vi "Remove Minor Frames.vi"(8 "error in (no error)":errorcluster, 10 "Minor Frame IDs":string[](array[string]), 11 "Major Frame in":refnum<class "Major Frame.lvclass">) -> (0 "error out":errorcluster, 3 "Major Frame out":refnum<class "Major Frame.lvclass">)   [LabVIEW 2020, in "BCI-1553 API.lvlib" / "Major Frame.lvclass"]
doc: "Removes a collection of Minor Frames from this Major Frame. These removed Minor Frames are no longer available to the Major Frame Schedule. The calling code must supply a new Schedule if the existing Schedule depends on a removed Minor Frame."
uses:
  Major Frame.lvclass
  Major Frame.lvclass/Major Frame.ctl
  Dependencies/Registry/Registry.lvclass/Registry.ctl
  Dependencies/Registry/Registry.lvclass
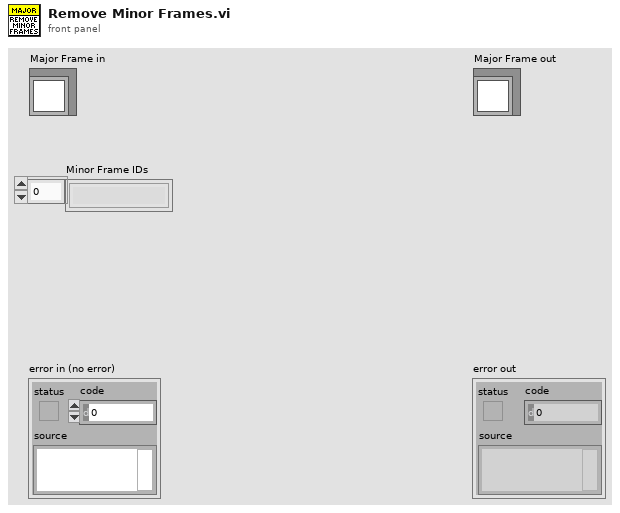
[diagram p1: front panel]
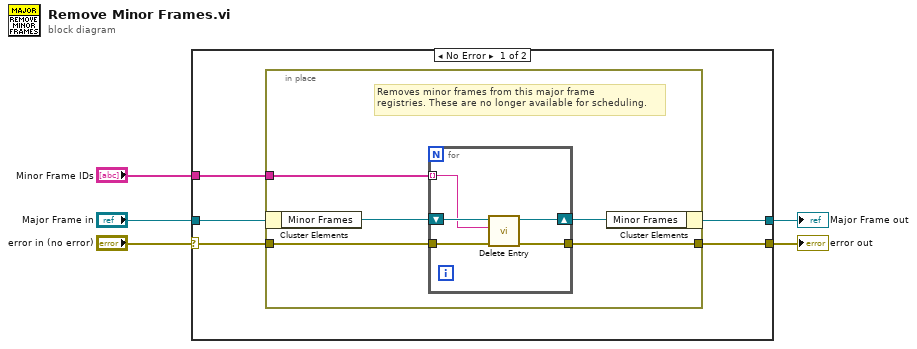
[diagram p0: block diagram]
diagram:
  n1 = case shown="No Error" "error in (no error)" {
    selector: "error in (no error)" -> [w7 w22]
    tunnel: [w8 w22] -> w3
    tunnel: [w9 w21] -> w2
    tunnel: "Major Frame in" -> [w10 w21]
    tunnel: "Minor Frame IDs" -> [w6 _]
    frame No Error {
      n2 = in-place {
        in-place-border: [w12] -> w8
        in-place-border: w7 -> [w14]
        in-place-border: w6 -> [w13]
        # "Removes minor frames from this major frame\nregistries. These are no longer available for scheduling."
        n3 = in-place-cluster #1(w10) -> ("Minor Frames"=w15:refnum<class "Registry.lvclass">)
        n4 = for {
          shift-right: [w17] -> w11
          shift-left: w15 -> [w20]
          tunnel: w14 -> [w19]
          tunnel: w13 -> [w18] mode=indexing
          tunnel: [w16] -> w12
          n5 = call "Delete Entry.vi"("error in (no error)"=w19, "Key"=w18, "Registry in"=w20) -> ("error out"=w16:errorcluster, "Registry out"=w17:refnum<class "Registry.lvclass">)  [unwired: 6 in, 1 out]
        }
        n6 = in-place-cluster #1("Minor Frames"=w11) -> (w9:refnum<class "Major Frame.lvclass">)
      }
    }
    frame Error {
    }
  }
  "error out" <- w3
  "Major Frame out" <- w2
